vi "acquiringTank1.vi"() -> ()   [LabVIEW 2012]
uses:
  <vilib>/imath/engines/lvmath2/RunTimeEngine/ErrorHandling/NIMS_Finalize Error.vi
  <vilib>/imath/engines/lvmath2/RunTimeEngine/BuiltInFunctions/size/NIMS_I32=size(GM,I32).vi
  <instcachedir>/0/NIMS_I32=size(GM,I32)_AF436776B5724EA8A5CFD6FACA63D3D9.lvgen/NIMS_I32=size(GM,I32)_AF436776B5724EA8A5CFD6FACA63D3D9_004.vi
  <vilib>/imathl/engines/lvmath/Functions/Error Handling/Create Error.vi
  <vilib>/imath/engines/lvmath2/RunTimeEngine/VariableToken/Read/NIMS_Get Elements - SorM(_,_) - Check - Check.vi
  <instcachedir>/0/NIMS_Get Elements - SorM(_,_) - Check - Check_3492346BAECA4EC09E2016EA7EC0034B.lvgen/NIMS_Get Elements - SorM(_,_) - Check - Check_3492346BAECA4EC09E2016EA7EC0034B_001.vi
  <vilib>/imath/engines/lvmath2/RunTimeEngine/NodeEndStatement/NIMS_NodeEndStatement_Output.vi
  <instcachedir>/0/NIMS_NodeEndStatement_Output_53EC0D466D134D7ABD903AC30B43404B.lvgen/NIMS_NodeEndStatement_Output_53EC0D466D134D7ABD903AC30B43404B_001.vi
  <instcachedir>/0/NIMS_NodeEndStatement_Output_53EC0D466D134D7ABD903AC30B43404B.lvgen/NIMS_NodeEndStatement_Output_53EC0D466D134D7ABD903AC30B43404B_013.vi
panel:
  out "Find":bool
  out "Numeric":dbl
  out "Angle":dbl(knob) scale=-35.0..35.0
  out "isNotGetten":bool
  out "Angle":dbl[][](array[numeric])
  in  "Stop (F)":bool
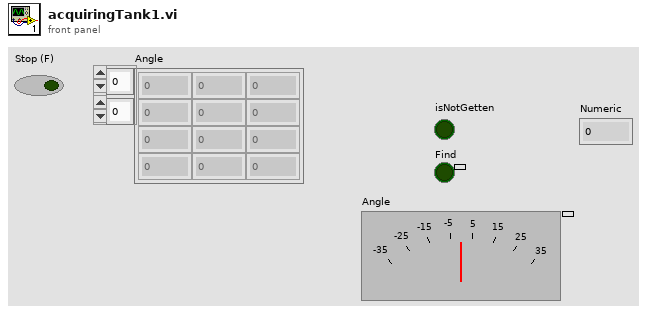
[diagram p1: front panel]
types:
  T1 = typedef "IMAQ Image.ctl" = refnum<image>
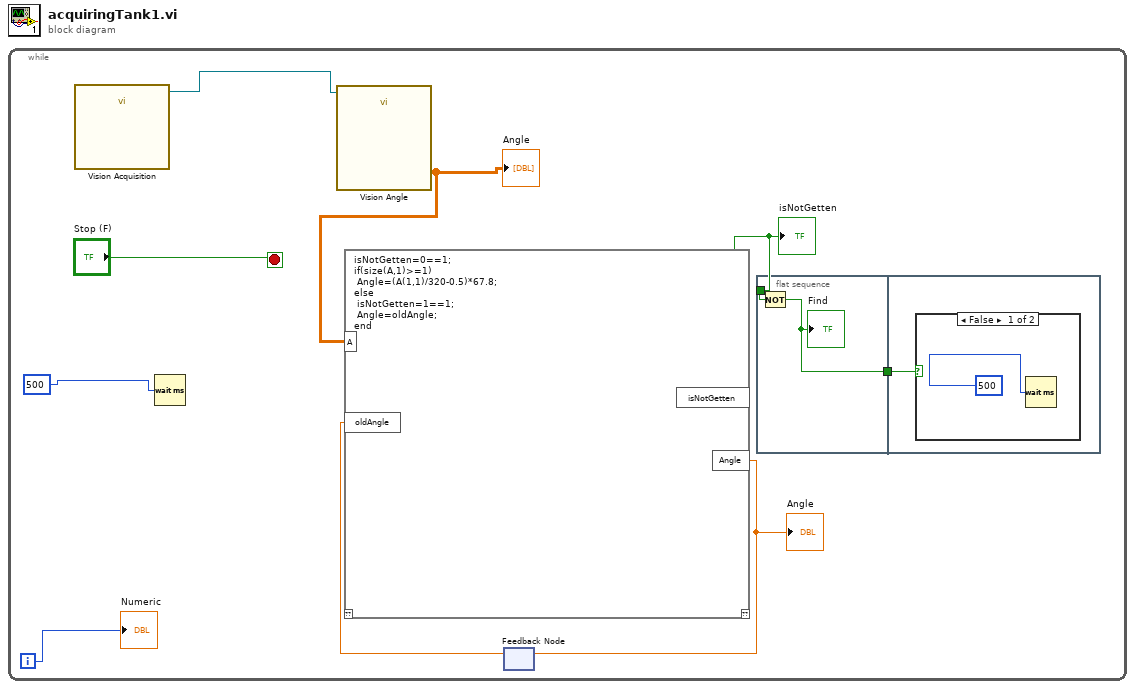
[diagram p0: block diagram]
diagram:
  n1 = while {
    i -> [w4]
    stop <- "Stop (F)" stop-if-true
    n2 = call "Vision Acquisition"() -> ("Image Out"=w9:T1)  [unwired: 25 in, 2 out]
    n3 = Wait (ms)(milliseconds to wait=500) -> ()  [unwired: 1 out]
    n4 = call "Vision Angle"("Image In"=w9) -> ("Particle Measurements (Pixels) (Particle Analysis 1)"=w7:dbl[][])  [unwired: 23 in, 3 out]
    "Angle" <- w7
    n5 = feedback #1() -> (w6:dbl)  [unwired: 1 in]
    n6 = mathscript code="isNotGetten=0==1;\nif(size(A,1)>=1)\n Angle=(A(1,1)/320-0.5)*67.8;\nelse\n isNotGetten=1==1;\n Angle=oldAngle;\nend"("A"=w7, "oldAngle"=w6) -> ("Angle"=w5:dbl, "isNotGetten"=w3:bool)  [unwired: 1 in, 1 out]
    "Angle" <- w5
    "isNotGetten" <- w3
    n7 = feedback-in #1(w5) -> ()
    n8 = flat-sequence {
      tunnel: w3 -> [w11]
      tunnel: [w10] -> w1
      tunnel: w1 -> [w12]
      frame #0 {
        n9 = Not(x=w11) -> (.not. x?=w10:bool)
        "Find" <- w10
      }
      frame #1 {
        n10 = case shown="False" w12 {
          frame False {
            n11 = Wait (ms)(milliseconds to wait=500) -> ()  [unwired: 1 out]
          }
          frame True {
          }
        }
      }
    }
    "Numeric" <- w4
  }
